vi "WriteProjectToController_Example.vi"(8 "Fehler (Eingang, kein Fehler)":errorcluster, 11 "Controller IP":string) -> (0 "Fehler (Ausgang)":errorcluster)   [LabVIEW 2016]
panel:
  out "ProjectID":string
  out "ConnectionToken":string
  out "ProjectPath":string
  out "State":string
  out "ControllerID":string
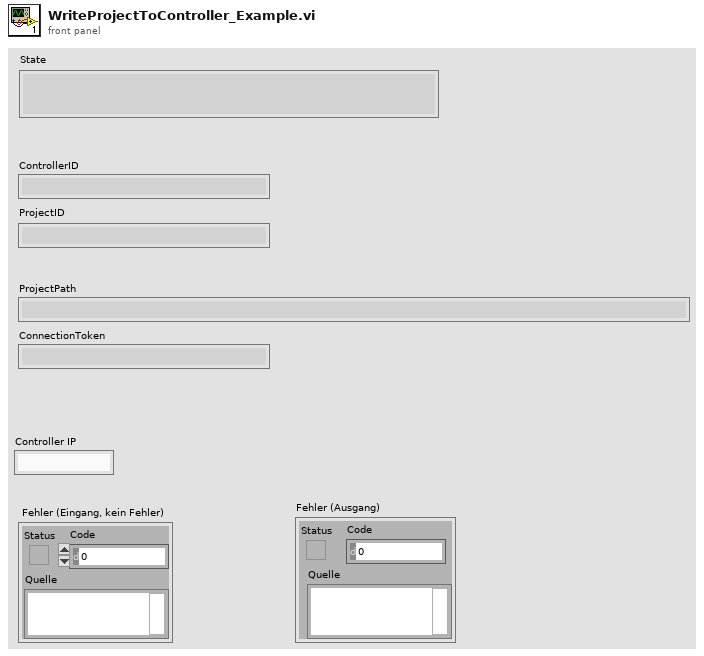
[diagram p1: front panel]
types:
  T1 = enum16{"Bool", "Snippet", "Struct", "Int64", "Int32", "Float", "Double", "String"}
  T2 = typedef "girpcutil_params.ctl" = cluster{"ConnectionHandle":i32, "DLL-Handle":cluster{"DLL Path":path, "Is32Bit":bool}}
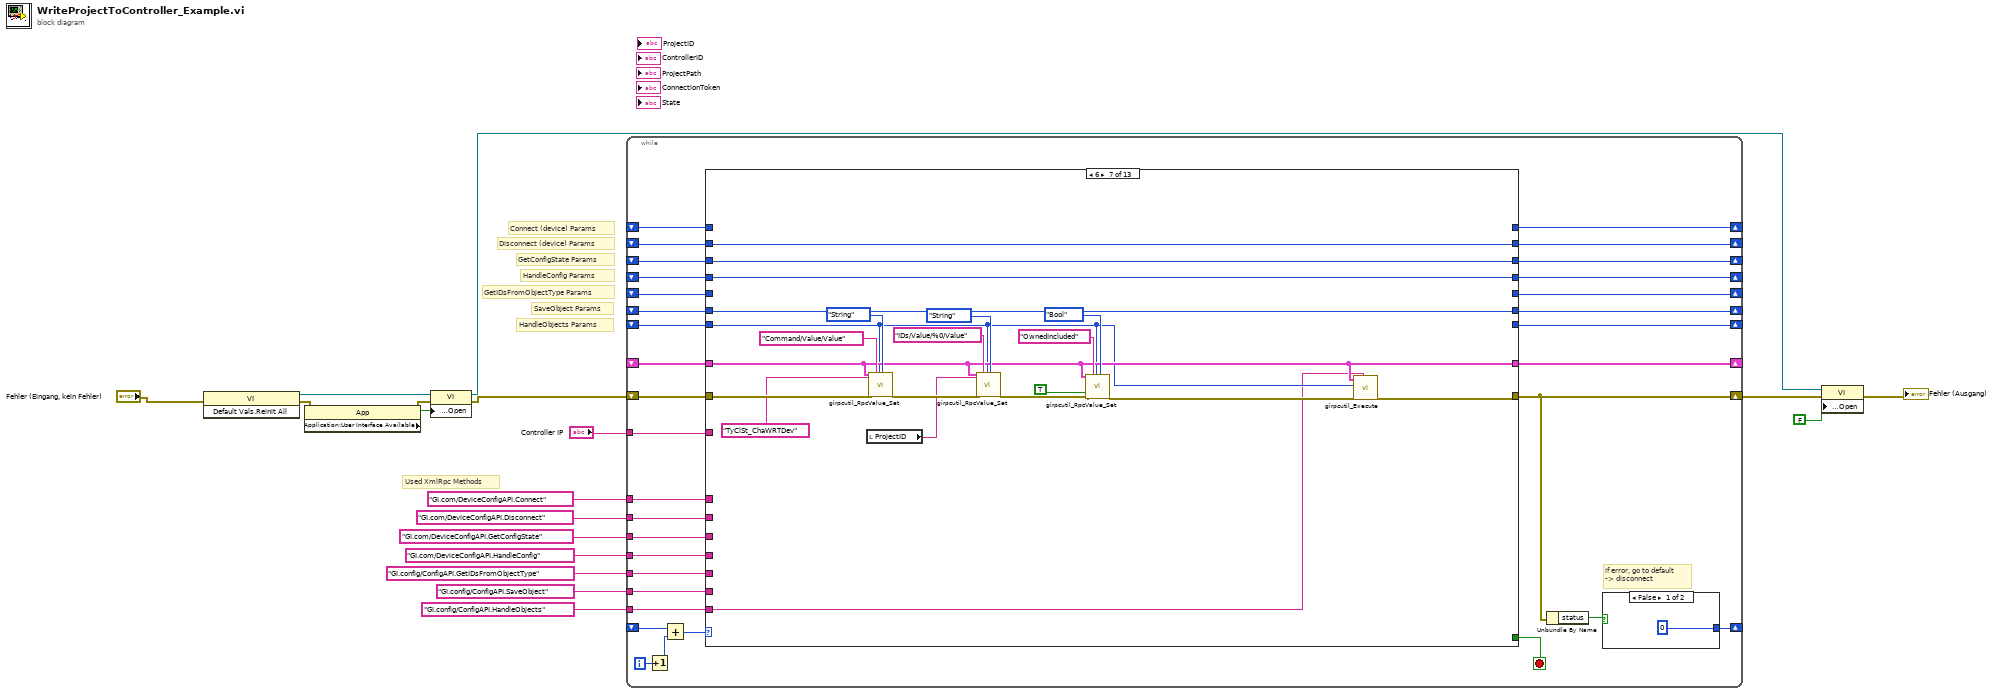
[diagram p0: block diagram]
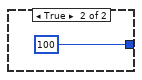
[diagram p2: hidden frame]
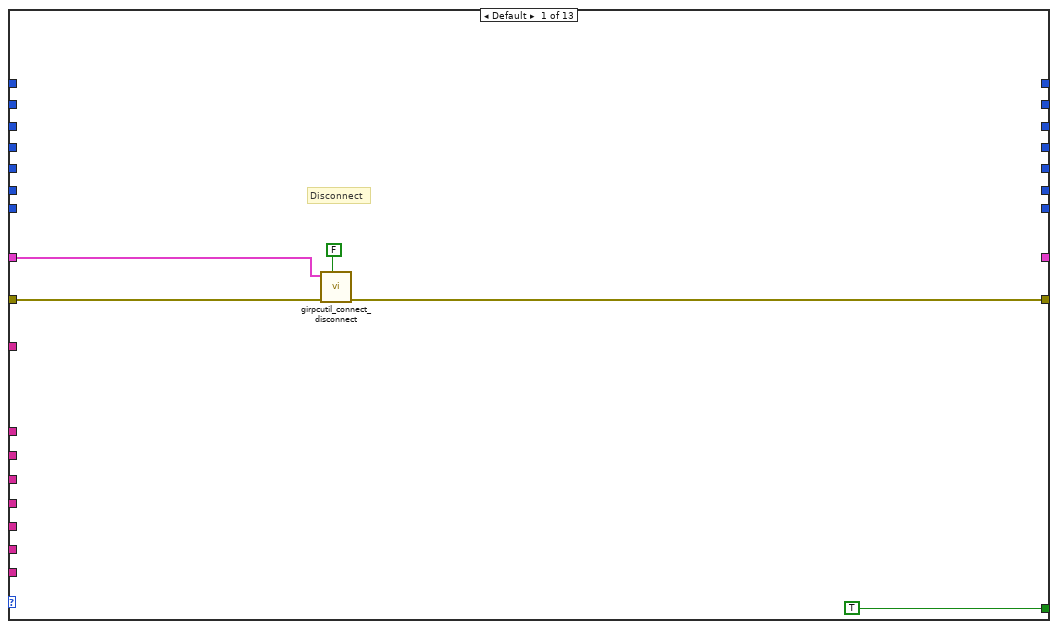
[diagram p3: hidden frame]
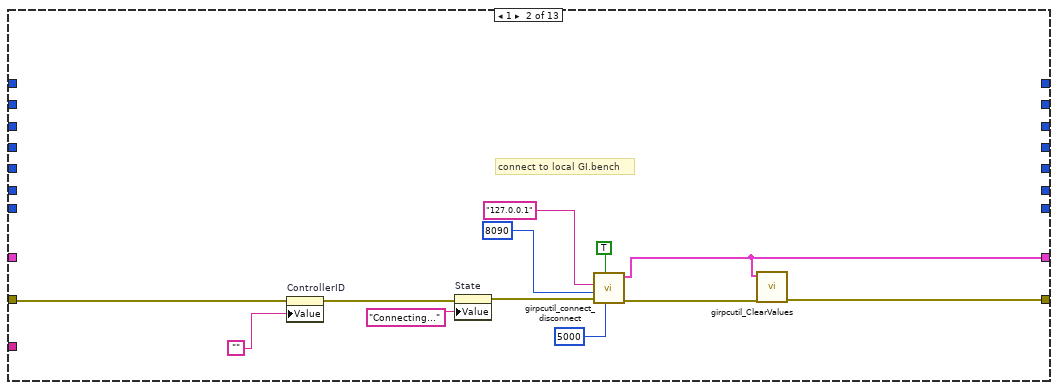
[diagram p4: hidden frame]
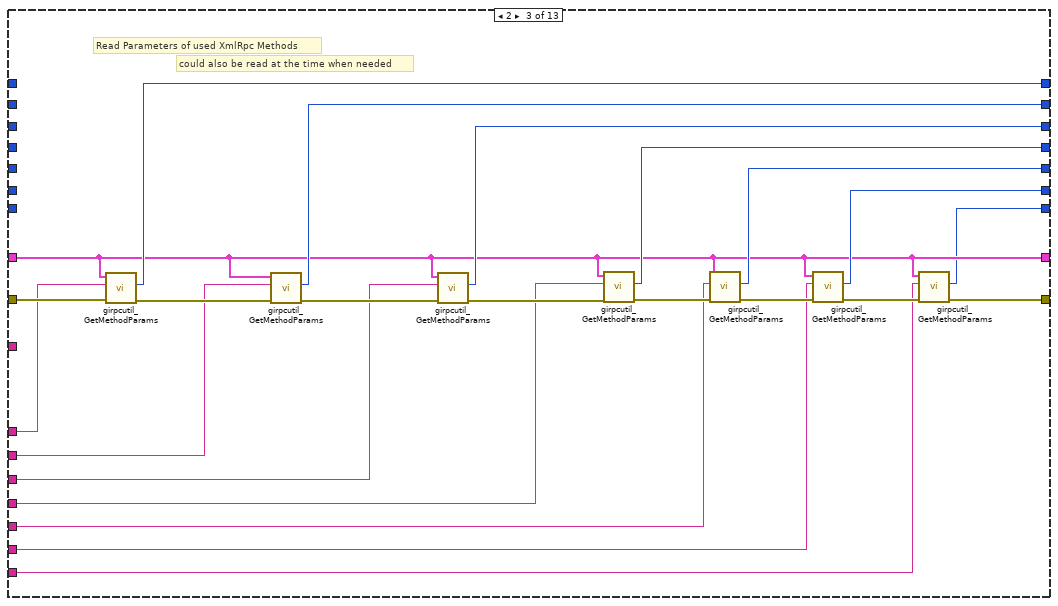
[diagram p5: hidden frame]
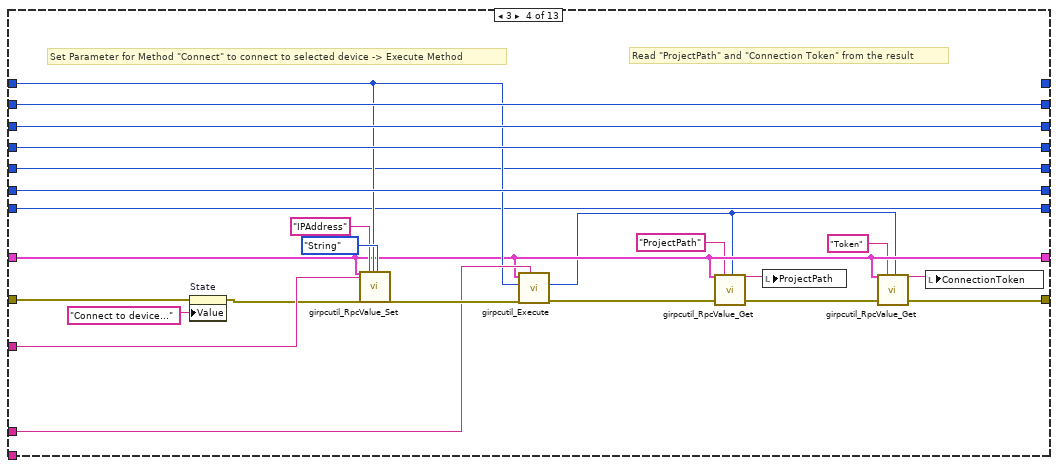
[diagram p6: hidden frame]
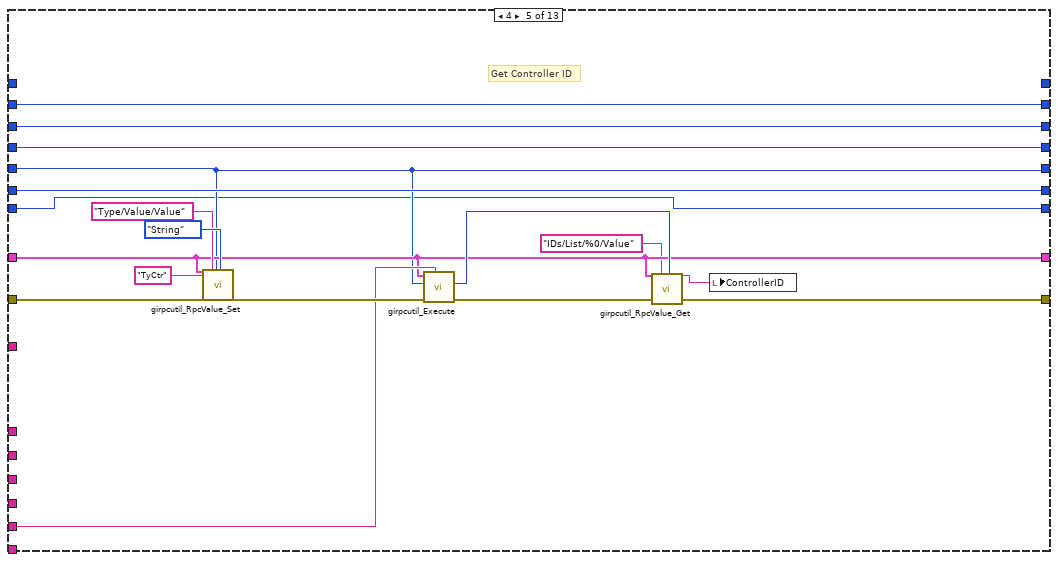
[diagram p7: hidden frame]
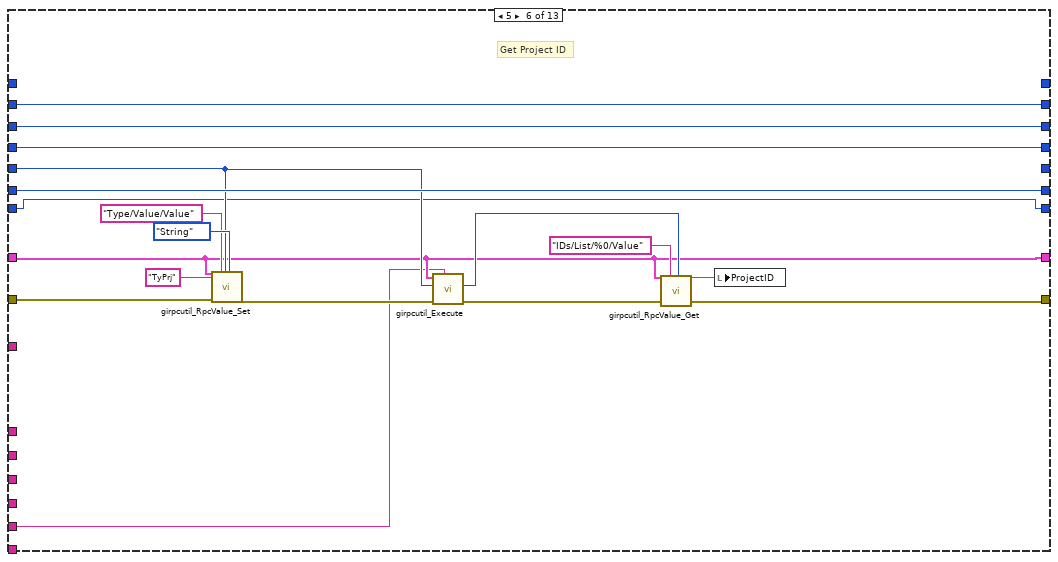
[diagram p8: hidden frame]
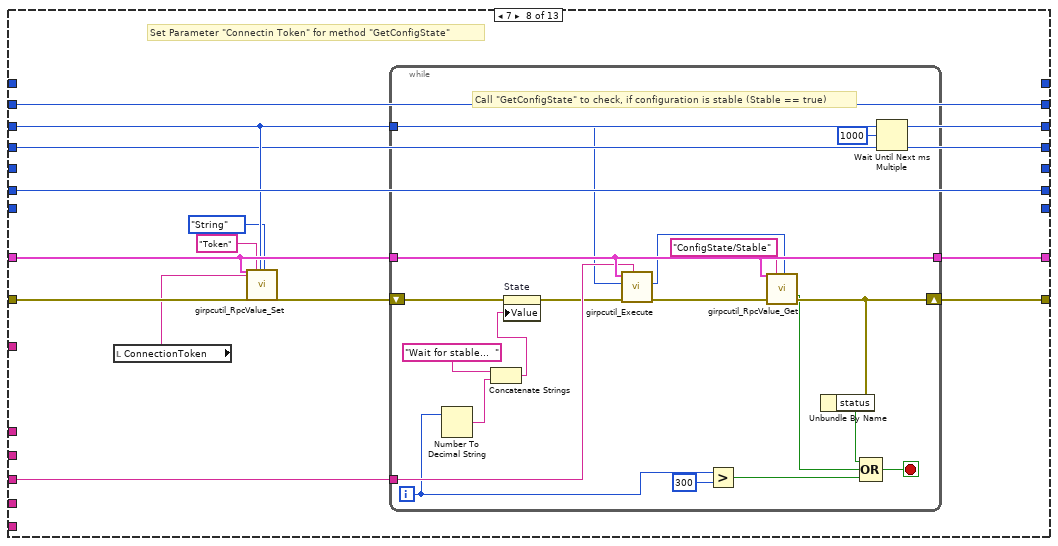
[diagram p9: hidden frame]
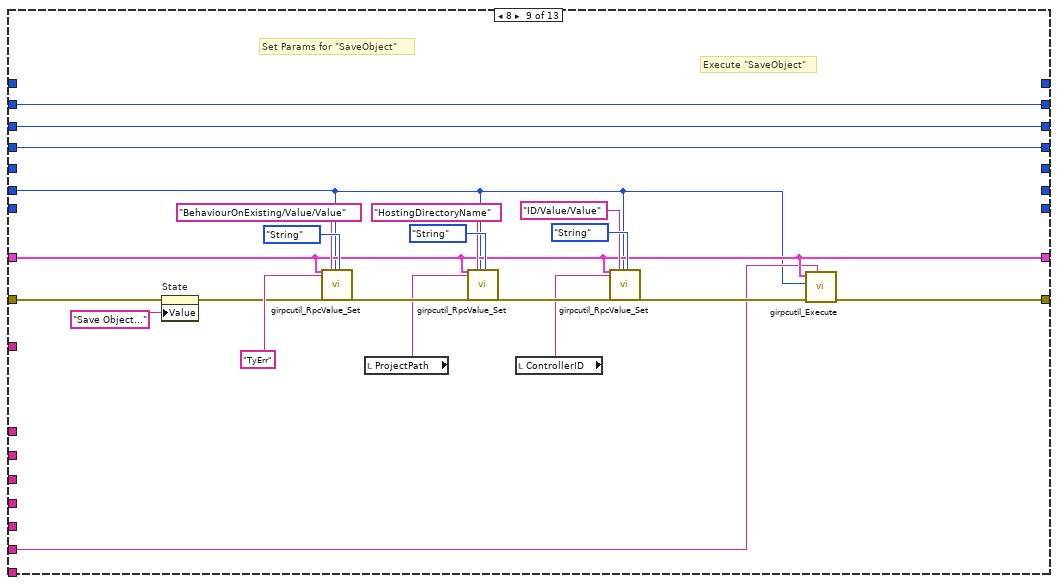
[diagram p10: hidden frame]
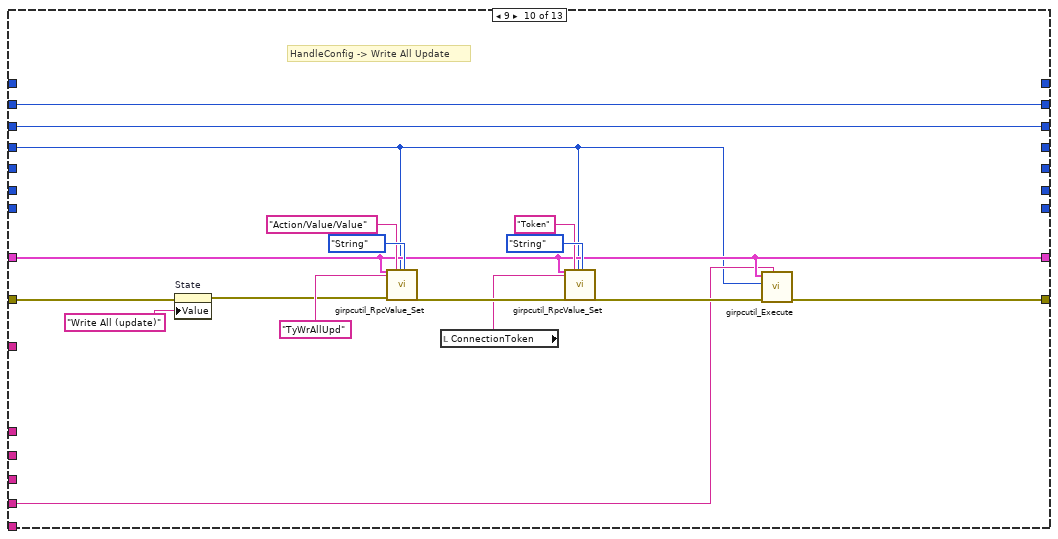
[diagram p11: hidden frame]
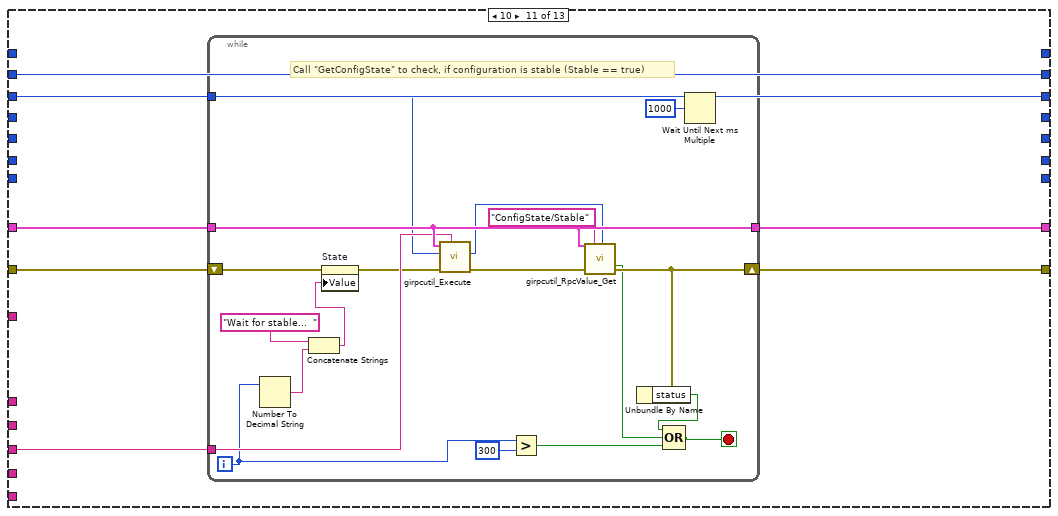
[diagram p12: hidden frame]
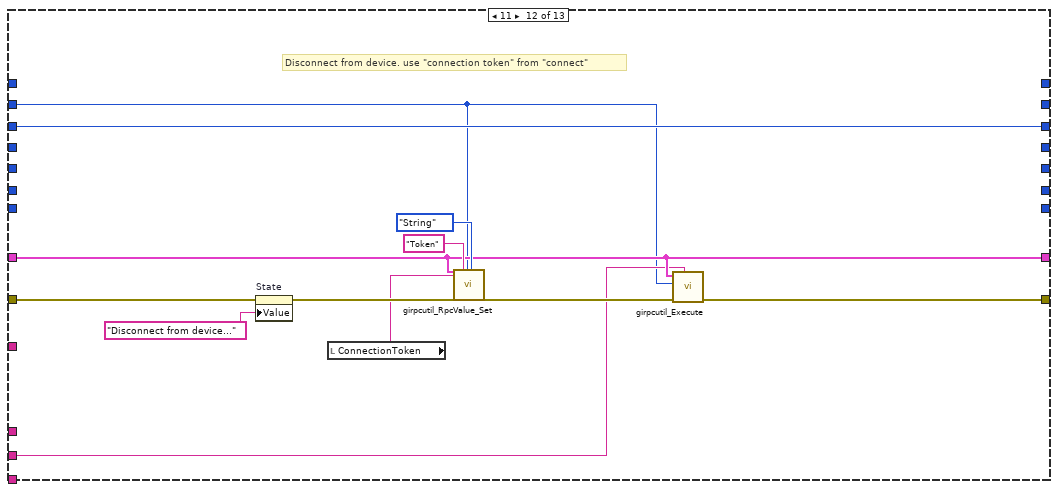
[diagram p13: hidden frame]
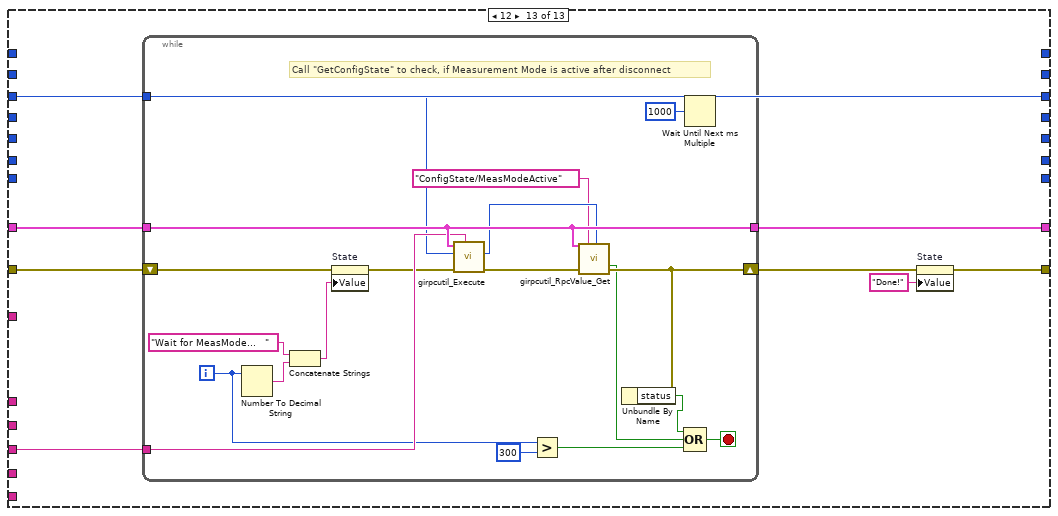
[diagram p14: hidden frame]
diagram:
  # "HandleObjects Params"
  # "SaveObject Params"
  # "GetIDsFromObjectType Params"
  # "HandleConfig Params"
  # "GetConfigState Params"
  # "Disconnect (device) Params"
  # "Connect (device) Params"
  # "Used XmlRpc Methods"
  n1 = invoke class="VI" method="Default Vals.Reinit All"(error in="Fehler (Eingang, kein Fehler)") -> (reference out=w11:refnum<vi>, error out=w9:errorcluster)  [unwired: 2 in, 1 out]
  n2 = property class="App"(error in=w9) -> (error out=w8:errorcluster, "Application:User Interface Available"=w10:bool)  [unwired: 1 in, 1 out]
  n3 = property class="VI"(reference=w11, error in=w8, "Front Panel.Open"=w10) -> (reference out=w2:refnum<vi>, error out=w6:errorcluster)
  n4 = while {
    shift-right: [w35] -> w4
    shift-left: w6 -> [w50]
    tunnel: "GI.com/DeviceConfigAPI.Connect" ("methodName") -> [w49]
    tunnel: "GI.com/DeviceConfigAPI.Disconnect" ("methodName") -> [w48]
    tunnel: "GI.com/DeviceConfigAPI.GetConfigState" ("methodName") -> [w47]
    tunnel: "GI.com/DeviceConfigAPI.HandleConfig" ("methodName") -> [w46]
    tunnel: "GI.config/ConfigAPI.GetIDsFromObjectType" ("methodName") -> [w45]
    tunnel: "GI.config/ConfigAPI.SaveObject" ("methodName") -> [w44]
    shift-right: [w43] -> _
    shift-left: _ -> [w42]
    shift-right: [w41] -> _
    shift-left: _ -> [w33]
    shift-right: [w40] -> _
    shift-left: _ -> [w32]
    shift-right: [w39] -> _
    shift-left: _ -> [w31]
    shift-right: [w38] -> _
    shift-left: _ -> [w30]
    shift-right: [w37] -> _
    shift-left: _ -> [w34]
    shift-right: [w36] -> _
    shift-left: _ -> [w29]
    shift-right: [w23] -> _
    shift-left: _ -> [w24]
    tunnel: "Controller IP" -> [w22]
    tunnel: "GI.config/ConfigAPI.HandleObjects" ("methodName") -> [w21]
    shift-right: [w20] -> _
    shift-left: _ -> [w19]
    i -> [w51]
    stop <- w28 stop-if-true
    # "if error, go to default\n-> disconnect"
    n5 = Increment(x=w51) -> (x+1=w26:i32)
    n6 = Add(x=w24, y=w26) -> (x+y=w25:i32)
    n7 = case shown="6" w25 {
      tunnel: [TRUE _ _ _ _ _ _ _ _ _ _ _ _] -> w28
      tunnel: w50 -> [w54 w61 w93 w99 w132 w142 w172 w182 w209 w231 w252 w274 w291]
      tunnel: [w57 w65 w74 w105 w121 w141 w161 w185 w213 w237 w251 w278 w285] -> w35
      tunnel: w49 -> [_ _ w87 w109 _ _ _ _ _ _ _ _ _]
      tunnel: w48 -> [_ _ w86 _ _ _ _ _ _ _ _ w279 _]
      tunnel: w47 -> [_ _ w85 _ _ _ _ w186 _ _ w246 _ w287]
      tunnel: w46 -> [_ _ w84 _ _ _ _ _ _ w235 _ _ _]
      tunnel: w45 -> [_ _ w83 _ w128 w143 _ _ _ _ _ _ _]
      tunnel: w44 -> [_ _ w82 _ _ _ _ _ w215 _ _ _ _]
      tunnel: [_ w64 w73 w104 w123 w144 w160 w187 w216 w236 w249 w280 w289] -> w43
      tunnel: w42 -> [w56 _ w73 w104 w123 w144 w160 w180 w216 w236 w250 w280 w290]
      tunnel: [_ _ w81 _ _ _ _ _ _ _ _ _ _] -> w41
      tunnel: [_ _ w80 w117 w135 w139 w157 w184 w212 w233 w247 _ _] -> w40
      tunnel: [_ _ w79 w116 w134 w138 w156 w179 w211 w232 w248 w277 w288] -> w39
      tunnel: [_ _ w78 w115 w127 w137 w155 w175 w210 _ _ _ _] -> w38
      tunnel: [_ _ w77 w95 w119 _ _ _ _ _ _ _ _] -> w37
      tunnel: [_ _ w76 w114 w126 w146 w154 w183 _ _ _ _ _] -> w36
      tunnel: w34 -> [_ _ _ w95 w119 w145 _ _ _ _ _ _ _]
      tunnel: w33 -> [_ _ _ w108 _ _ _ _ _ _ _ _ _]
      tunnel: w32 -> [_ _ _ w117 w135 w139 w157 w184 w212 w233 w247 w276 _]
      tunnel: w31 -> [_ _ _ w116 w134 w138 w156 w179 w211 w232 w248 w277 w288]
      tunnel: w30 -> [_ _ _ w115 w127 w137 w155 w175 w210 w234 _ _ _]
      tunnel: w29 -> [_ _ _ w114 w126 w146 w154 w183 w214 _ _ _ _]
      tunnel: w22 -> [_ _ _ w111 _ _ _ _ _ _ _ _ _]
      tunnel: w21 -> [_ _ w72 _ _ _ w158 _ _ _ _ _ _]
      tunnel: [_ _ w71 w94 w118 w136 _ _ _ _ _ _ _] -> w20
      tunnel: w19 -> [_ _ _ w94 w118 w136 w159 _ _ _ _ _ _]
      frame Default {
        # "Disconnect"
        n8 = call "girpcutil_connect_disconnect.vi"("Connect"=FALSE, "Fehler (Eingang, kein Fehler)"=w54, "girpcutil_params"=w56) -> ("Fehler (Ausgang)"=w57:errorcluster)  [unwired: 7 in, 1 out]
      }
      frame 1 {
        # "connect to local GI.bench"
        n9 = property on="ControllerID" class="Str"(error in=w61, "Value"="") -> (error out=w60:errorcluster)  [unwired: 1 in, 1 out]
        n10 = property on="State" class="Str"(error in=w60, "Value"="Connecting..." ("State")) -> (error out=w63:errorcluster)  [unwired: 1 in, 1 out]
        n11 = call "girpcutil_connect_disconnect.vi"("timeout"=u32 5000, "Connect"=TRUE, "Fehler (Eingang, kein Fehler)"=w63, "port"=u32 8090, "host"="127.0.0.1") -> ("Fehler (Ausgang)"=w66:errorcluster, "girpcutil_params 2"=w64:T2)  [unwired: 5 in]
        n12 = call "girpcutil_ClearValues.vi"("Fehler (Eingang, kein Fehler)"=w66, "girpcutil_params"=w64) -> ("error IO"=w65:errorcluster)  [unwired: 9 in]
      }
      frame 2 {
        # "could also be read at the time when needed"
        # "Read Parameters of used XmlRpc Methods"
        n13 = call "girpcutil_GetMethodParams.vi"("Fehler (Eingang, kein Fehler)"=w93, "methodName"=w87, "girpcutil_params"=w73) -> ("Fehler (Ausgang)"=w92:errorcluster, "param handle out"=w81:i32)  [unwired: 7 in]
        n14 = call "girpcutil_GetMethodParams.vi"("Fehler (Eingang, kein Fehler)"=w92, "methodName"=w86, "girpcutil_params"=w73) -> ("Fehler (Ausgang)"=w91:errorcluster, "param handle out"=w80:i32)  [unwired: 7 in]
        n15 = call "girpcutil_GetMethodParams.vi"("Fehler (Eingang, kein Fehler)"=w91, "methodName"=w85, "girpcutil_params"=w73) -> ("Fehler (Ausgang)"=w90:errorcluster, "param handle out"=w79:i32)  [unwired: 7 in]
        n16 = call "girpcutil_GetMethodParams.vi"("Fehler (Eingang, kein Fehler)"=w90, "methodName"=w84, "girpcutil_params"=w73) -> ("Fehler (Ausgang)"=w89:errorcluster, "param handle out"=w78:i32)  [unwired: 7 in]
        n17 = call "girpcutil_GetMethodParams.vi"("Fehler (Eingang, kein Fehler)"=w89, "methodName"=w83, "girpcutil_params"=w73) -> ("Fehler (Ausgang)"=w88:errorcluster, "param handle out"=w77:i32)  [unwired: 7 in]
        n18 = call "girpcutil_GetMethodParams.vi"("Fehler (Eingang, kein Fehler)"=w88, "methodName"=w82, "girpcutil_params"=w73) -> ("Fehler (Ausgang)"=w75:errorcluster, "param handle out"=w76:i32)  [unwired: 7 in]
        n19 = call "girpcutil_GetMethodParams.vi"("Fehler (Eingang, kein Fehler)"=w75, "methodName"=w72, "girpcutil_params"=w73) -> ("Fehler (Ausgang)"=w74:errorcluster, "param handle out"=w71:i32)  [unwired: 7 in]
      }
      frame 3 {
        # "Read \"ProjectPath\" and \"Connection Token\" from the result"
        # "Set Parameter for Method \"Connect\" to connect to selected device -> Execute Method"
        n20 = property on="State" class="Str"(error in=w99, "Value"="Connect to device..." ("State")) -> (error out=w98:errorcluster)  [unwired: 1 in, 1 out]
        n21 = call "girpcutil_RpcValue_Set.vi"("girpcutil_params"=w104, "StringValue or Snippet"=w111, "Fehler (Eingang, kein Fehler)"=w98, "MemberName"="IPAddress", "param handle"=w108, "DataType"=T1."String") -> ("Fehler (Ausgang)"=w110:errorcluster)  [unwired: 21 in]
        n22 = call "girpcutil_Execute.vi"("methodName"=w109, "Fehler (Eingang, kein Fehler)"=w110, "params"=w108, "girpcutil_params"=w104) -> ("Fehler (Ausgang)"=w106:errorcluster, "results"=w103:i32)  [unwired: 6 in]
        n23 = call "girpcutil_RpcValue_Get.vi"("girpcutil_params"=w104, "Fehler (Eingang, kein Fehler)"=w106, "member"="ProjectPath", "value"=w103) -> ("StringResult"=w97:string, "Fehler (Ausgang)"=w107:errorcluster)  [unwired: 19 in, 3 out]
        n24 = local write "ProjectPath"(w97) -> ()
        n25 = call "girpcutil_RpcValue_Get.vi"("girpcutil_params"=w104, "Fehler (Eingang, kein Fehler)"=w107, "member"="Token", "value"=w103) -> ("StringResult"=w96:string, "Fehler (Ausgang)"=w105:errorcluster)  [unwired: 19 in, 3 out]
        n26 = local write "ConnectionToken"(w96) -> ()
      }
      frame 4 {
        # "Get Controller ID"
        n27 = call "girpcutil_RpcValue_Set.vi"("girpcutil_params"=w123, "StringValue or Snippet"="TyCtr", "Fehler (Eingang, kein Fehler)"=w132, "MemberName"="Type/Value/Value", "param handle"=w119, "DataType"=T1."String") -> ("Fehler (Ausgang)"=w129:errorcluster)  [unwired: 21 in]
        n28 = call "girpcutil_Execute.vi"("methodName"=w128, "Fehler (Eingang, kein Fehler)"=w129, "params"=w119, "girpcutil_params"=w123) -> ("Fehler (Ausgang)"=w125:errorcluster, "results"=w124:i32)  [unwired: 6 in]
        n29 = call "girpcutil_RpcValue_Get.vi"("girpcutil_params"=w123, "Fehler (Eingang, kein Fehler)"=w125, "member"="IDs/List/%0/Value", "value"=w124) -> ("StringResult"=w120:string, "Fehler (Ausgang)"=w121:errorcluster)  [unwired: 19 in, 3 out]
        n30 = local write "ControllerID"(w120) -> ()
      }
      frame 5 {
        # "Get Project ID"
        n31 = call "girpcutil_RpcValue_Set.vi"("girpcutil_params"=w144, "StringValue or Snippet"="TyPrj", "Fehler (Eingang, kein Fehler)"=w142, "MemberName"="Type/Value/Value", "param handle"=w145, "DataType"=T1."String") -> ("Fehler (Ausgang)"=w150:errorcluster)  [unwired: 21 in]
        n32 = call "girpcutil_Execute.vi"("methodName"=w143, "Fehler (Eingang, kein Fehler)"=w150, "params"=w145, "girpcutil_params"=w144) -> ("Fehler (Ausgang)"=w149:errorcluster, "results"=w148:i32)  [unwired: 6 in]
        n33 = call "girpcutil_RpcValue_Get.vi"("girpcutil_params"=w144, "Fehler (Eingang, kein Fehler)"=w149, "member"="IDs/List/%0/Value", "value"=w148) -> ("StringResult"=w140:string, "Fehler (Ausgang)"=w141:errorcluster)  [unwired: 19 in, 3 out]
        n34 = local write "ProjectID"(w140) -> ()
      }
      frame 6 {
        n35 = local read "ProjectID"() -> (w167:string)
        n36 = call "girpcutil_RpcValue_Set.vi"("girpcutil_params"=w160, "StringValue or Snippet"="TyClSt_ChaWRTDev", "Fehler (Eingang, kein Fehler)"=w172, "MemberName"="Command/Value/Value", "param handle"=w159, "DataType"=T1."String") -> ("Fehler (Ausgang)"=w170:errorcluster)  [unwired: 21 in]
        n37 = call "girpcutil_RpcValue_Set.vi"("girpcutil_params"=w160, "StringValue or Snippet"=w167, "Fehler (Eingang, kein Fehler)"=w170, "MemberName"="IDs/Value/%0/Value", "param handle"=w159, "DataType"=T1."String") -> ("Fehler (Ausgang)"=w166:errorcluster)  [unwired: 21 in]
        n38 = call "girpcutil_RpcValue_Set.vi"("girpcutil_params"=w160, "BoolValue"=TRUE, "Fehler (Eingang, kein Fehler)"=w166, "MemberName"="OwnedIncluded", "param handle"=w159, "DataType"=T1."Bool") -> ("Fehler (Ausgang)"=w162:errorcluster)  [unwired: 21 in]
        n39 = call "girpcutil_Execute.vi"("methodName"=w158, "Fehler (Eingang, kein Fehler)"=w162, "params"=w159, "girpcutil_params"=w160) -> ("Fehler (Ausgang)"=w161:errorcluster)  [unwired: 6 in, 1 out]
      }
      frame 7 {
        # "Set Parameter \"Connectin Token\" for method \"GetConfigState\""
        n40 = local read "ConnectionToken"() -> (w176:string)
        n41 = call "girpcutil_RpcValue_Set.vi"("girpcutil_params"=w180, "StringValue or Snippet"=w176, "Fehler (Eingang, kein Fehler)"=w182, "MemberName"="Token", "param handle"=w179, "DataType"=T1."String") -> ("Fehler (Ausgang)"=w181:errorcluster)  [unwired: 21 in]
        n42 = while {
          shift-right: [w198] -> w185
          shift-left: w181 -> [w197]
          tunnel: w180 -> [w205]
          tunnel: [w205] -> w187
          tunnel: w186 -> [w204]
          tunnel: w179 -> [w203]
          i -> [w190]
          stop <- w199 stop-if-true
          # "Call \"GetConfigState\" to check, if configuration is stable (Stable == true)"
          n43 = Number To Decimal String(number=w190) -> (decimal integer string=w193:string)  [unwired: 1 in]
          n44 = Concatenate Strings("Wait for stable...  " ("State"), w193) -> (w194:string)
          n45 = property on="State" class="Str"(error in=w197, "Value"=w194) -> (error out=w196:errorcluster)  [unwired: 1 in, 1 out]
          n46 = call "girpcutil_Execute.vi"("methodName"=w204, "Fehler (Eingang, kein Fehler)"=w196, "params"=w203, "girpcutil_params"=w205) -> ("Fehler (Ausgang)"=w206:errorcluster, "results"=w202:i32)  [unwired: 6 in]
          n47 = Greater?(x=w190, y=300) -> (0:w188:bool)
          n48 = call "girpcutil_RpcValue_Get.vi"("girpcutil_params"=w205, "Fehler (Eingang, kein Fehler)"=w206, "member"="ConfigState/Stable", "value"=w202) -> ("BoolResult"=w191:bool, "Fehler (Ausgang)"=w198:errorcluster)  [unwired: 19 in, 3 out]
          n49 = Unbundle By Name(w198) -> ("status"=w192:bool)
          n50 = Compound Arithmetic op=OR(w192, w191, w188) -> (w199:bool)
          n51 = Wait Until Next ms Multiple(millisecond multiple=u32 1000) -> ()  [unwired: 1 out]
        }
      }
      frame 8 {
        # "Execute \"SaveObject\""
        # "Set Params for \"SaveObject\""
        n52 = property on="State" class="Str"(error in=w209, "Value"="Save Object..." ("State")) -> (error out=w208:errorcluster)  [unwired: 1 in, 1 out]
        n53 = call "girpcutil_RpcValue_Set.vi"("girpcutil_params"=w216, "StringValue or Snippet"="TyErr", "Fehler (Eingang, kein Fehler)"=w208, "MemberName"="BehaviourOnExisting/Value/Value", "param handle"=w214, "DataType"=T1."String") -> ("Fehler (Ausgang)"=w225:errorcluster)  [unwired: 21 in]
        n54 = local read "ProjectPath"() -> (w219:string)
        n55 = call "girpcutil_RpcValue_Set.vi"("girpcutil_params"=w216, "StringValue or Snippet"=w219, "Fehler (Eingang, kein Fehler)"=w225, "MemberName"="HostingDirectoryName", "param handle"=w214, "DataType"=T1."String") -> ("Fehler (Ausgang)"=w224:errorcluster)  [unwired: 21 in]
        n56 = local read "ControllerID"() -> (w220:string)
        n57 = call "girpcutil_RpcValue_Set.vi"("girpcutil_params"=w216, "StringValue or Snippet"=w220, "Fehler (Eingang, kein Fehler)"=w224, "MemberName"="ID/Value/Value", "param handle"=w214, "DataType"=T1."String") -> ("Fehler (Ausgang)"=w217:errorcluster)  [unwired: 21 in]
        n58 = call "girpcutil_Execute.vi"("methodName"=w215, "Fehler (Eingang, kein Fehler)"=w217, "params"=w214, "girpcutil_params"=w216) -> ("Fehler (Ausgang)"=w213:errorcluster)  [unwired: 6 in, 1 out]
      }
      frame 9 {
        # "HandleConfig -> Write All Update"
        n59 = property on="State" class="Str"(error in=w231, "Value"="Write All (update)" ("State")) -> (error out=w230:errorcluster)  [unwired: 1 in, 1 out]
        n60 = call "girpcutil_RpcValue_Set.vi"("girpcutil_params"=w236, "StringValue or Snippet"="TyWrAllUpd", "Fehler (Eingang, kein Fehler)"=w230, "MemberName"="Action/Value/Value", "param handle"=w234, "DataType"=T1."String") -> ("Fehler (Ausgang)"=w240:errorcluster)  [unwired: 21 in]
        n61 = local read "ConnectionToken"() -> (w239:string)
        n62 = call "girpcutil_RpcValue_Set.vi"("girpcutil_params"=w236, "StringValue or Snippet"=w239, "Fehler (Eingang, kein Fehler)"=w240, "MemberName"="Token", "param handle"=w234, "DataType"=T1."String") -> ("Fehler (Ausgang)"=w238:errorcluster)  [unwired: 21 in]
        n63 = call "girpcutil_Execute.vi"("methodName"=w235, "Fehler (Eingang, kein Fehler)"=w238, "params"=w234, "girpcutil_params"=w236) -> ("Fehler (Ausgang)"=w237:errorcluster)  [unwired: 6 in, 1 out]
      }
      frame 10 {
        n64 = while {
          shift-right: [w264] -> w251
          shift-left: w252 -> [w263]
          tunnel: w250 -> [w270]
          tunnel: [w270] -> w249
          tunnel: w246 -> [w269]
          tunnel: w248 -> [w268]
          i -> [w253]
          stop <- w256 stop-if-true
          # "Call \"GetConfigState\" to check, if configuration is stable (Stable == true)"
          n65 = Number To Decimal String(number=w253) -> (decimal integer string=w259:string)  [unwired: 1 in]
          n66 = Concatenate Strings("Wait for stable...  " ("State"), w259) -> (w260:string)
          n67 = property on="State" class="Str"(error in=w263, "Value"=w260) -> (error out=w262:errorcluster)  [unwired: 1 in, 1 out]
          n68 = call "girpcutil_Execute.vi"("methodName"=w269, "Fehler (Eingang, kein Fehler)"=w262, "params"=w268, "girpcutil_params"=w270) -> ("Fehler (Ausgang)"=w271:errorcluster, "results"=w267:i32)  [unwired: 6 in]
          n69 = Greater?(x=w253, y=300) -> (0:w257:bool)
          n70 = call "girpcutil_RpcValue_Get.vi"("girpcutil_params"=w270, "Fehler (Eingang, kein Fehler)"=w271, "member"="ConfigState/Stable", "value"=w267) -> ("BoolResult"=w254:bool, "Fehler (Ausgang)"=w264:errorcluster)  [unwired: 19 in, 3 out]
          n71 = Unbundle By Name(w264) -> ("status"=w255:bool)
          n72 = Compound Arithmetic op=OR(w255, w254, w257) -> (w256:bool)
          n73 = Wait Until Next ms Multiple(millisecond multiple=u32 1000) -> ()  [unwired: 1 out]
        }
      }
      frame 11 {
        # "Disconnect from device. use \"connection token\" from \"connect\""
        n74 = property on="State" class="Str"(error in=w274, "Value"="Disconnect from device..." ("State")) -> (error out=w273:errorcluster)  [unwired: 1 in, 1 out]
        n75 = local read "ConnectionToken"() -> (w272:string)
        n76 = call "girpcutil_RpcValue_Set.vi"("girpcutil_params"=w280, "StringValue or Snippet"=w272, "Fehler (Eingang, kein Fehler)"=w273, "MemberName"="Token", "param handle"=w276, "DataType"=T1."String") -> ("Fehler (Ausgang)"=w281:errorcluster)  [unwired: 21 in]
        n77 = call "girpcutil_Execute.vi"("methodName"=w279, "Fehler (Eingang, kein Fehler)"=w281, "params"=w276, "girpcutil_params"=w280) -> ("Fehler (Ausgang)"=w278:errorcluster)  [unwired: 6 in, 1 out]
      }
      frame 12 {
        n78 = while {
          shift-right: [w303] -> w286
          shift-left: w291 -> [w302]
          tunnel: w290 -> [w309]
          tunnel: [w309] -> w289
          tunnel: w287 -> [w308]
          tunnel: w288 -> [w307]
          i -> [w292]
          stop <- w295 stop-if-true
          # "Call \"GetConfigState\" to check, if Measurement Mode is active after disconnect"
          n79 = Number To Decimal String(number=w292) -> (decimal integer string=w298:string)  [unwired: 1 in]
          n80 = Concatenate Strings("Wait for MeasMode...   " ("State"), w298) -> (w299:string)
          n81 = property on="State" class="Str"(error in=w302, "Value"=w299) -> (error out=w301:errorcluster)  [unwired: 1 in, 1 out]
          n82 = call "girpcutil_Execute.vi"("methodName"=w308, "Fehler (Eingang, kein Fehler)"=w301, "params"=w307, "girpcutil_params"=w309) -> ("Fehler (Ausgang)"=w310:errorcluster, "results"=w306:i32)  [unwired: 6 in]
          n83 = Greater?(x=w292, y=300) -> (0:w296:bool)
          n84 = call "girpcutil_RpcValue_Get.vi"("girpcutil_params"=w309, "Fehler (Eingang, kein Fehler)"=w310, "member"="ConfigState/MeasModeActive", "value"=w306) -> ("BoolResult"=w293:bool, "Fehler (Ausgang)"=w303:errorcluster)  [unwired: 19 in, 3 out]
          n85 = Unbundle By Name(w303) -> ("status"=w294:bool)
          n86 = Compound Arithmetic op=OR(w294, w293, w296) -> (w295:bool)
          n87 = Wait Until Next ms Multiple(millisecond multiple=u32 1000) -> ()  [unwired: 1 out]
        }
        n88 = property on="State" class="Str"(error in=w286, "Value"="Done!" ("State")) -> (error out=w285:errorcluster)  [unwired: 1 in, 1 out]
      }
    }
    n89 = Unbundle By Name(w35) -> ("status"=w27:bool)
    n90 = case shown="False" w27 {
      tunnel: [0 100] -> w23
      frame False {
      }
      frame True {
      }
    }
  }
  n91 = property class="VI"(reference=w2, error in=w4, "Front Panel.Open"=FALSE ("Frontpanel-Fenster:Öffnen")) -> (error out=→"Fehler (Ausgang)":errorcluster)  [unwired: 1 out]
